vi "sinswave.vi"() -> ()   [LabVIEW 2016]
uses:
  <vilib>/Utility/file.llb/Write Delimited Spreadsheet (DBL).vi
  <vilib>/Utility/file.llb/Read Delimited Spreadsheet (DBL).vi
  <vilib>/measure/NI_MABase.lvlib
panel:
  out "Waveform Graph":dynamicdata(graph)
  in  "m(t)":T1(ring)
  in  "Stop Button":bool
  in  "A":dbl=1.0 format="%0.2p"
  in  "freq":dbl=10.0 format="%0.2p"
  in  "?":T1(ring)
  in  "sampling info":cluster{"Fs":dbl, "#s":dbl}={"Fs"=1000.0, "#s"=1000.0} {"Fs" format="%.2p"}
  in  "phase":dbl format="%.2p"
  in  "K":dbl=1.0 format="%0.2p"
  in  "f0":dbl=10.0 format="%0.2p"
  # "s(t)= m(t) * (1 + k * sin(2pi * f0 * t + phase ))\n\n\nm(t)= A * sin (2pi * freq * t)"
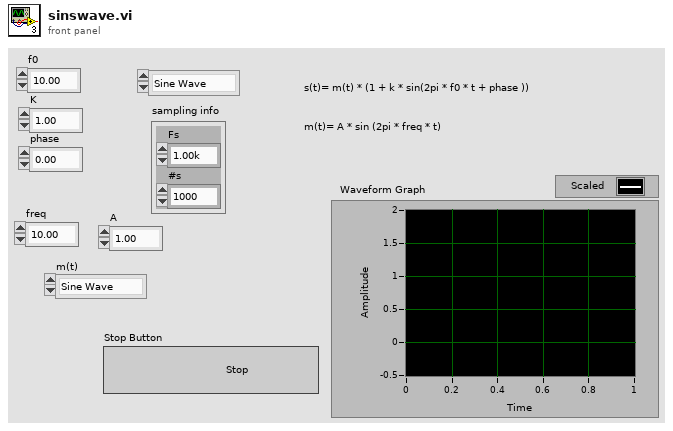
[diagram p1: front panel]
types:
  T1 = enum16{"Sine Wave", "Triangle Wave", "Square Wave", "Sawtooth Wave"}
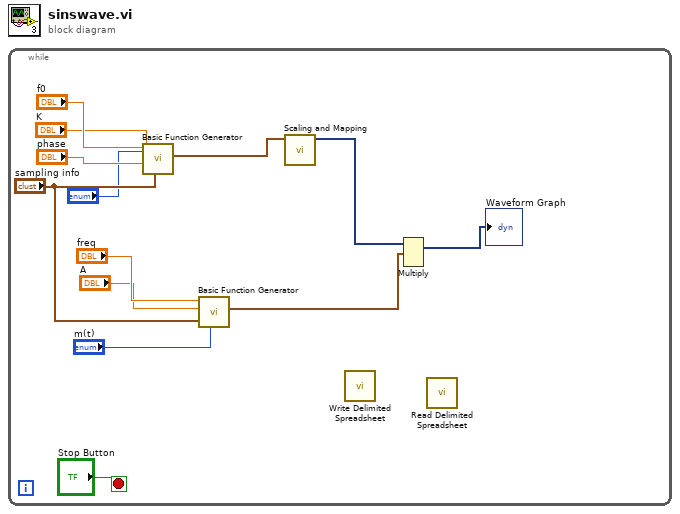
[diagram p0: block diagram]
diagram:
  n1 = while {
    stop <- "Stop Button" stop-if-true
    n2 = call <vilib>:"Basic Function Generator.vi"("sampling info"="sampling info", "signal type"="?", "phase"="phase", "amplitude"="K", "frequency"="f0") -> ("signal out"=w4:waveform(dbl))  [unwired: 4 in, 2 out]
    n3 = call <vilib>:"Basic Function Generator.vi"("sampling info"="sampling info", "signal type"="m(t)", "amplitude"="A", "frequency"="freq") -> ("signal out"=w2:waveform(dbl))  [unwired: 5 in, 2 out]
    n4 = call "Scaling and Mapping"("Signals"=w4) -> ("Scaled Signals"=w3:dynamicdata)  [unwired: 9 in, 1 out]
    n5 = call-poly <vilib>:"Write Delimited Spreadsheet.vi"() -> ()  [unwired: 14 in, 2 out]
    n6 = Multiply(1:w2, 2:w3) -> (0:→"Waveform Graph":dynamicdata)  [unwired: 1 in, 1 out]
    n7 = call-poly <vilib>:"Read Delimited Spreadsheet.vi"() -> ()  [unwired: 10 in, 6 out]
  }
